vi "LVClass_HasoSlopes ctor from dimension.vi"(0 "HasoSlopes in":refnum<class "HasoSlopes.lvclass">, 5 "Dimensions_um":T1, 7 "serial":string, 11 "error in (no error)":errorcluster) -> (4 "HasoSlopes out":refnum<class "HasoSlopes.lvclass">, 15 "error out":errorcluster)   [LabVIEW 2020, in "HasoSlopes.lvclass"]
doc: "HasoSlopes constructor from dimensions and steps.\n\n--------------------------------------------------------------------------------\n\n<B>HasoSlopesIn </B> : Constant Pointer to HasoSlopes object.\n<B>HasoSlopesOut </B> : Constant Pointer to HasoSlopes object.\n<B>size </B> : 2D subpupils number of the HasoSlopes.\n<B>step </B> : 2D step of subpupils.\n<B>serial_number </B> : Serial number.\n<B>ErrorIn </B> : Error\n<B>ErrorOut </B> : Error\n\n--------------------------------------------------------------------------------"
uses:
  HasoSlopes.lvclass
  General dimensions definition.ctl
  Point2D.ctl
  Point2Df.ctl
  Handle creation.ctl
  HasoSlopes.lvclass/HasoSlopes.ctl
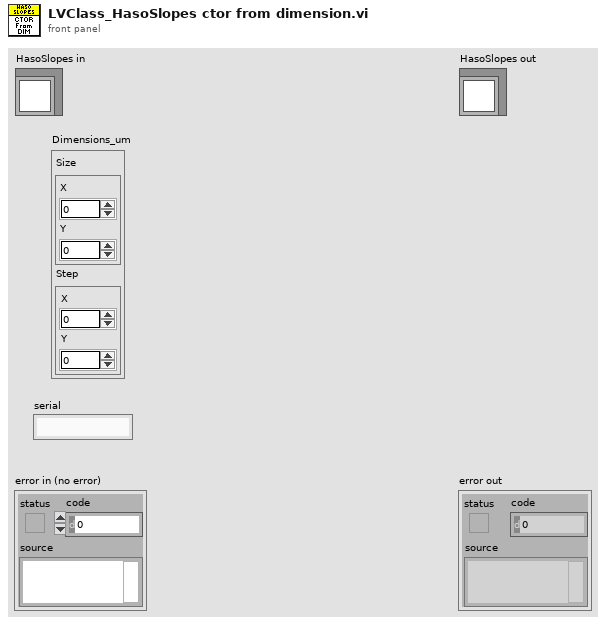
[diagram p1: front panel]
types:
  T1 = typedef "General dimensions definition.ctl" = cluster{"Size":T2, "Step":T3}
  T2 = typedef "Point2D.ctl" = cluster{"X":u32, "Y":u32}
  T3 = typedef "Point2Df.ctl" = cluster{"X":sgl, "Y":sgl}
  T4 = typedef "Handle creation.ctl" = enum16{"By ctor", "By write function"}
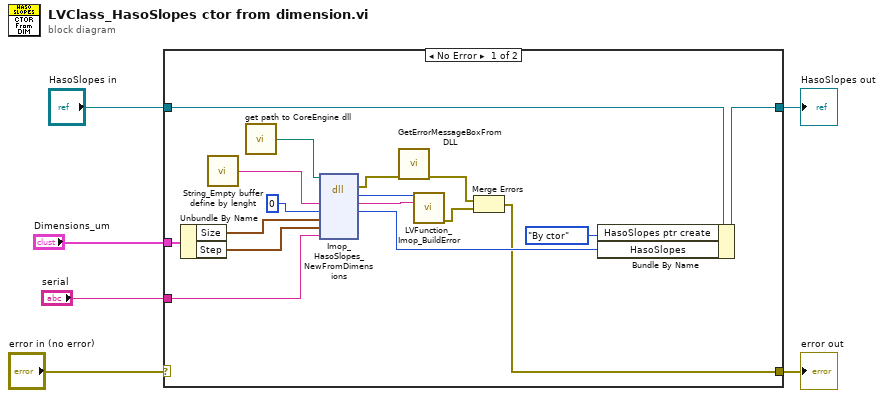
[diagram p0: block diagram]
diagram:
  n1 = case shown="No Error" "error in (no error)" {
    selector: "error in (no error)" -> [_ w25]
    tunnel: [w8 w25] -> w5
    tunnel: [w17 w24] -> w4
    tunnel: "HasoSlopes in" -> [w18 w24]
    tunnel: "Dimensions_um" -> [w13 _]
    tunnel: "serial" -> [w7 _]
    frame No Error {
      n2 = Unbundle By Name(w13) -> ("Size"=w12:T2, "Step"=w11:T3)
      n3 = call "String_Empty buffer define by lenght.vi"() -> ("Empty buffer"=w19:string)  [unwired: 1 in]
      n4 = call "get path to CoreEngine dll.vi"() -> ("path to c_interface_vc100.dll"=w16:path)  [unwired: 12 in, 3 out]
      n5 = dll-call lib="D:/soft/HASO_v3/SVN_trunk/ImOpCoreEngine4_LV2011/DLLs/c_interface_vc100.dll" fn="Imop_HasoSlopes_NewFromDimensions"(path in=w16, "message"=w19, "objet"=0, "size"=w12, "step"=w11, "serial"=w7) -> (error out=w15:errorcluster, "return type"=w22:i32, "message"=w21:string, "objet"=w20:i32)  [unwired: 5 in, 1 out]
      n6 = call "GetErrorMessageBoxFromDLL.vi"("error IN"=w15) -> ("error OUT"=w10:errorcluster)  [unwired: 10 in]
      n7 = call "LVFunction_Imop_BuildError.vi"("code"=w22, "String to Prepend to source (\"\")"=w21) -> ("error out"=w9:errorcluster)  [unwired: 13 in]
      n8 = Merge Errors(w10, w9) -> (w8:errorcluster)
      n9 = Bundle By Name(cluster=w18, "HasoSlopes ptr create"=Handle_creation."By ctor", "HasoSlopes"=w20) -> (w17:refnum<class "HasoSlopes.lvclass">)
    }
    frame Error {
    }
  }
  "error out" <- w5
  "HasoSlopes out" <- w4
